vi "FTW-JSON-Core-LibraryFilepath.vi"(8 "error in":errorcluster, 10 "Rediscover library?":bool) -> (0 "error out":errorcluster, 2 "JSON Library Filepath":path)   [LabVIEW 2013]
uses:
  FTWLib-Jansson-Win32.dll
  FTWLib-Jansson-Win64.dll
  FTWLib-Jansson-LinuxRT.so
panel:
  # "Inputs"
  # "Outputs"
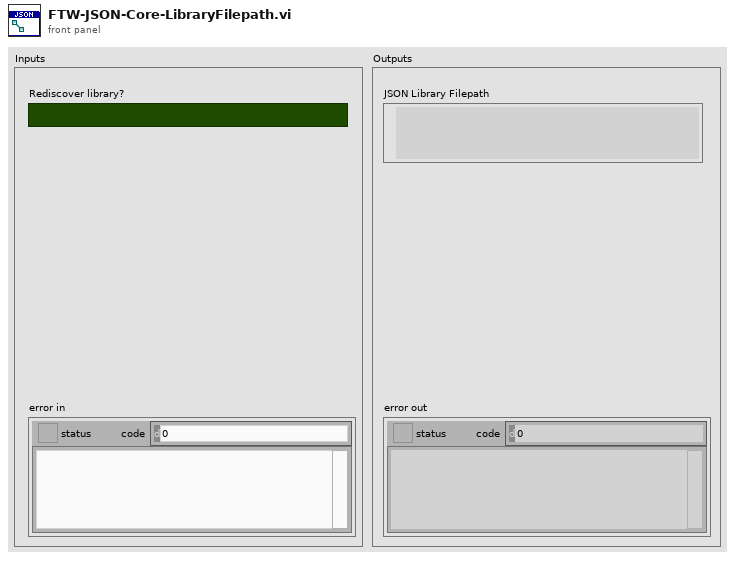
[diagram p1: front panel]
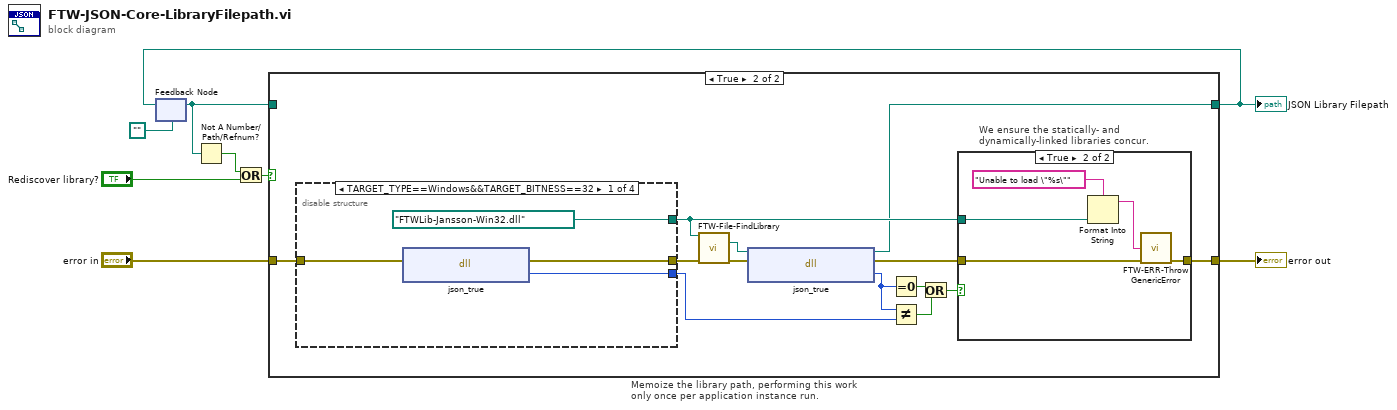
[diagram p0: block diagram]
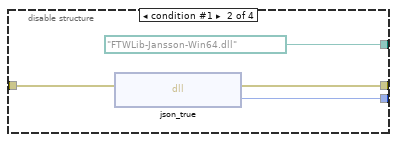
[diagram p4: hidden frame]
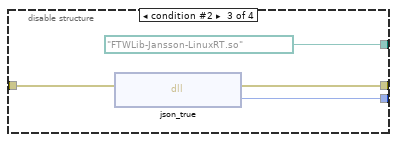
[diagram p5: hidden frame]
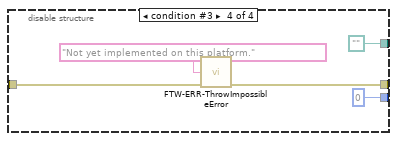
[diagram p6: hidden frame]
diagram:
  n1 = feedback #1(path "") -> (w2:path)
  n2 = Not A Number/Path/Refnum?(number/path/refnum=w2) -> (NaN/Path/Refnum?=w1:bool)
  n3 = Or(x=w1, y="Rediscover library?") -> (x .or. y?=w4:bool)
  n4 = case "Memoize the library path, performing this work only once per application instance run." shown="True" w4 {
    tunnel: [w10 w15] -> w6
    tunnel: "error in" -> [w9 w23]
    tunnel: [w9 w20] -> w7
    tunnel: w2 -> [w10 _]
    frame False {
    }
    frame True {
      n5 = disable-structure shown="TARGET_TYPE==Windows&&TARGET_BITNESS==32" {
        disable-tunnel: [path "FTWLib-Jansson-Win32.dll" path "FTWLib-Jansson-Win64.dll" path "FTWLib-Jansson-LinuxRT.so" path ""] -> w19
        disable-tunnel: [w31 w36 w39 w45] -> w22
        disable-tunnel: w23 -> [w32 w37 w41 w46]
        disable-tunnel: [w30 w34 w38 i64 0 ("True Constant Pointer")] -> w21
        frame condition #0 (active) {
          n6 = dll-call lib="C:/Users/Jack/repo/ftw-master/Core/src/JSON/FTWLib-Jansson-Win32.dll" fn="json_true" label="FTWLib-Jansson-Win32.dll"(error in=w32) -> (error out=w31:errorcluster, "True Constant Pointer"=w30:i64)  [unwired: 2 in, 1 out]
        }
        frame condition #1 {
          n7 = dll-call lib="C:/Users/Jack/repo/ftw-master/Core/src/JSON/FTWLib-Jansson-Win64.dll" fn="json_true" label="FTWLib-Jansson-Win64.dll"(error in=w37) -> (error out=w36:errorcluster, "True Constant Pointer"=w34:i64)  [unwired: 2 in, 1 out]
        }
        frame condition #2 {
          n8 = dll-call lib="C:/Users/Jack/repo/ftw-master/Core/src/JSON/FTWLib-Jansson-LinuxRT.so" fn="json_true" label="FTWLib-Jansson-LinuxRT.so"(error in=w41) -> (error out=w39:errorcluster, "True Constant Pointer"=w38:i64)  [unwired: 2 in, 1 out]
        }
        frame condition #3 {
          n9 = call "FTW-ERR-ThrowImpossibleError.vi"("Reason this error should never happen"="Not yet implemented on this platform.", "error in"=w46) -> ("error out"=w45:errorcluster)  [unwired: 13 in]
        }
      }
      n10 = call "FTW-File-FindLibrary.vi"("Library File Pattern"=w19, "error in"=w22) -> ("Library Filepath"=w18:path, "error out"=w17:errorcluster)  [unwired: 12 in]
      n11 = dll-call lib="?" fn="json_true"(path in=w18, error in=w17) -> (path out=w15:path, error out=w16:errorcluster, "True Constant Pointer"=w14:i64)  [unwired: 1 in]
      n12 = Equal To 0?(x=w14) -> (x = 0?=w13:bool)
      n13 = Not Equal?(x=w14, y=w21) -> (x != y?=w12:bool)
      n14 = Or(x=w13, y=w12) -> (x .or. y?=w11:bool)
      n15 = case "We ensure the statically- and\ndynamically-linked libraries concur." shown="True" w11 {
        tunnel: w16 -> [w24 w29]
        tunnel: [w24 w28] -> w20
        tunnel: w19 -> [_ w27]
        frame False {
        }
        frame True {
          n16 = Format Into String(format string="Unable to load \"%s\"", w27) -> (resulting string=w26:string)  [unwired: 2 in, 1 out]
          n17 = call "FTW-ERR-ThrowGenericError.vi"("Error Message"=w26, "error in"=w29) -> ("error out"=w28:errorcluster)  [unwired: 13 in]
        }
      }
    }
  }
  "error out" <- w7
  "JSON Library Filepath" <- w6
  n18 = feedback-in #1(w6) -> ()
